vi "Spawn Message Handler.vi"(7 "Base Server":refnum<class "Server.lvclass">, 8 "error in (no error)":errorcluster, 10 "WebSocket in":refnum<class "WebSocket.lvclass">, 11 "Message Handler in":refnum<class "Handler.lvclass">) -> (0 "error out":errorcluster)   [LabVIEW 2024, in "Ramses Framework.lvlib" / "Handler.lvclass"]
uses:
  Handler.lvclass
  <vilib>/MediaMongrels Ltd/WebSockets/WebSockets/WebSocket/WebSocket.lvclass
  Base Server/Server.lvclass
  Handler.lvclass/Handler.ctl
  Handle Specific Message.vi
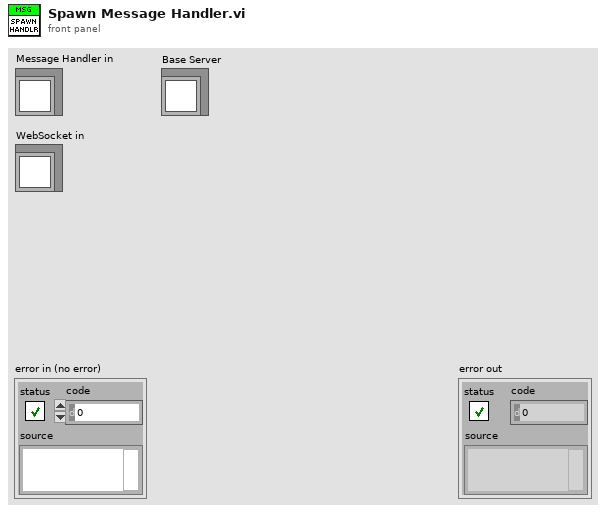
[diagram p1: front panel]
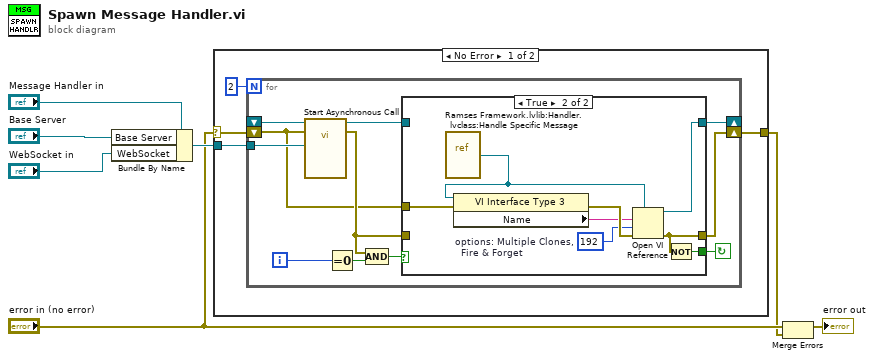
[diagram p0: block diagram]
diagram:
  n1 = Bundle By Name(cluster="Message Handler in", "Base Server"="Base Server", "WebSocket"="WebSocket in") -> (w4:refnum<class "Handler.lvclass">)
  n2 = case shown="No Error" "error in (no error)" {
    selector: "error in (no error)" -> [w8 w33]
    tunnel: w4 -> [w11 _]
    tunnel: [w9 w33] -> w1
    frame No Error {
      n3 = for {
        N: 2 -> [_]
        tunnel: w11 -> [w22]
        shift-right: [w21] -> _
        shift-left: _ -> [w20]
        shift-right: [w18] -> w9
        shift-left: w8 -> [w12]
        i -> [w15]
        stop <- w13 continue-if-true
        n4 = call-by-ref "Start Asynchronous Call"(reference=w20, error in=w12, "Handler in"=w22) -> (reference out=w19:refnum<vi>, error out=w14:errorcluster)  [unwired: 11 in]
        n5 = Equal To 0?(x=w15) -> (x = 0?=w16:bool)
        n6 = Compound Arithmetic op=AND(w14, w16) -> (w17:bool)
        n7 = case shown="True" w17 {
          tunnel: [w24 w29] -> w21
          tunnel: [w23 w27] -> w18
          tunnel: w19 -> [w24 _]
          tunnel: w14 -> [w23 _]
          tunnel: [_ w28] -> w13
          tunnel: w12 -> [_ w26]
          frame False {
          }
          frame True {
            w30 = 192  # options: Multiple Clones,   Fire & Forget
            n8 = vi-ref "Ramses Framework.lvlib:Handler.lvclass:Handle Specific Message.vi"() -> (w25:refnum<vi>)
            n9 = property class="VI Interface Type 3"(reference=w25, error in=w26) -> (error out=w32:errorcluster, "Name"=w31:string)  [unwired: 1 out]
            n10 = Open VI Reference(type specifier VI Refnum (for type only)=w25, vi path=w31, options=w30, error in (no error)=w32) -> (vi reference=w29:refnum<vi>, error out=w27:errorcluster)  [unwired: 2 in]
            n11 = Not(x=w27) -> (.not. x?=w28:bool)
          }
        }
      }
    }
    frame Error {
    }
  }
  n12 = Merge Errors("error in (no error)", w1) -> (→"error out":errorcluster)
